vi "Find Project Target Item By VI.vi"(8 "vi name":string, 11 "project":refnum<vi>) -> (0 "found":bool, 3 "TargetItem Refnum":refnum<vi>)   [LabVIEW 2020, in "NI_TargetHelper.lvlib"]
uses:
  <vilib>/TargetSupport/NI_TargetHelper/NI_TargetHelper.lvlib
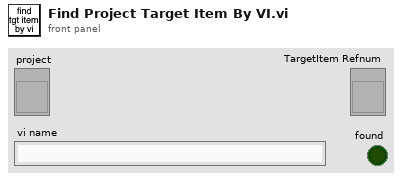
[diagram p1: front panel]
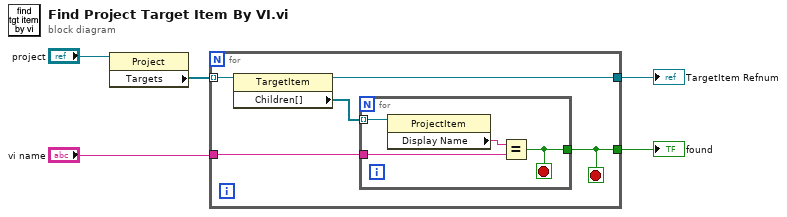
[diagram p0: block diagram]
diagram:
  n1 = property class="Project"(reference="project") -> ("Targets"=w5:refnum<vi>[])  [unwired: 1 in, 2 out]
  n2 = for {
    tunnel: w5 -> [w10] mode=indexing
    tunnel: "vi name" -> [w7]
    tunnel: [w9] -> w3
    tunnel: [w6] -> w2
    stop <- w6 stop-if-true
    n3 = property class="TargetItem"(reference=w10) -> (reference out=w9:refnum<vi>, "Children[]"=w8:refnum<vi>[])  [unwired: 1 in, 1 out]
    n4 = for {
      tunnel: w8 -> [w14] mode=indexing
      tunnel: w7 -> [w12]
      tunnel: [w11] -> w6
      stop <- w11 stop-if-true
      n5 = property class="ProjectItem"(reference=w14) -> ("Display Name"=w13:string)  [unwired: 1 in, 2 out]
      n6 = Equal?(x=w13, y=w12) -> (x = y?=w11:bool)
    }
  }
  "TargetItem Refnum" <- w3
  "found" <- w2
